vi "Axis_Go Related.vi"(10 "Distance":dbl format="%#_13g", 11 "Axis Index":i32) -> (0 "error":errorcluster)   [LabVIEW 2019]
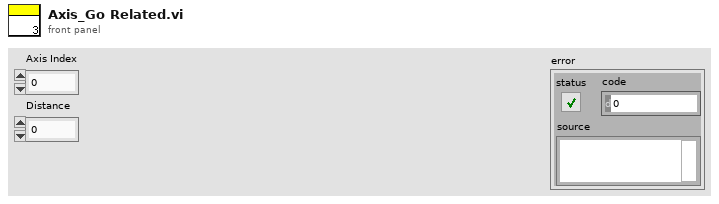
[diagram p1: front panel]
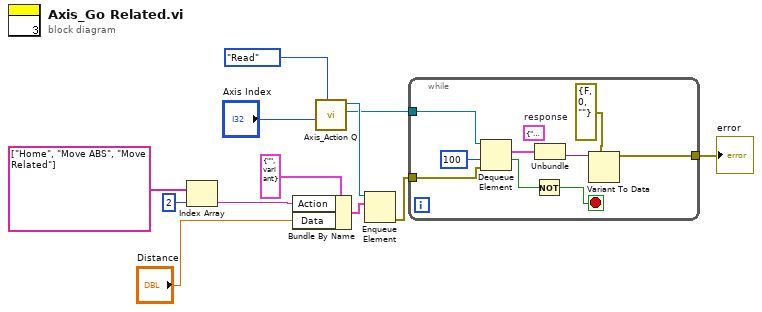
[diagram p0: block diagram]
diagram:
  n1 = Index Array(array=string[] ["Home", "Move ABS", "Move Related"], index=2) -> (element=w6:string)
  n2 = Bundle By Name(cluster=cluster{"Action":string, "Data":variant} {"Action"="", "Data"=variant} ("element"), "Action"=w6, "Data"="Distance") -> (w7:cluster{"Action":string, "Data":variant})
  n3 = call "Axis_Action Q.vi"("Enum"=enum16{"Initial", "Write", "Read"}."Read", "Axis Index"="Axis Index") -> ("Axis ActFeedBackQ Out"=w4:refnum<queue>, "Axis ActQ Out"=w10:refnum<queue>)  [unwired: 7 in, 1 out]
  n4 = Enqueue Element(queue=w10, element=w7) -> (error out=w3:errorcluster)  [unwired: 2 in, 2 out]
  n5 = while {
    tunnel: w4 -> [w21]
    tunnel: w3 -> [w20]
    tunnel: [w13] -> w2
    stop <- w16 stop-if-true
    (unwired) cluster{"Result":string, "error":errorcluster} {"Result"="", "error"={"status"=FALSE, "code"=0, "source"=""}}  # response
    n6 = Dequeue Element(queue=w21, timeout in ms (-1)=100, error in (no error)=w20) -> (element=w18:cluster{"Action":string, "Data":variant}, timed out?=w17:bool)  [unwired: 2 out]
    n7 = Not(x=w17) -> (.not. x?=w16:bool)
    n8 = Unbundle(w18) -> ("Data"=w15:variant)  [unwired: 1 out]
    n9 = Variant To Data(type=errorcluster {"status"=FALSE, "code"=0, "source"=""} ("error constant"), Variant=w15) -> (data=w13:errorcluster)  [unwired: 1 in, 1 out]
  }
  "error" <- w2
